vi "LabViewSLOTMACHINEFINAL.vi"() -> ()   [LabVIEW 2025]
panel:
  out "Bet info":string
  in  "stop":bool
  out "Minor Prize":bool
  out "Major Prize":bool
  out "Grand Prize":bool
  out "Array of Nums":dbl[](array[numeric])
  out "Balance Info":string
  out "Balance":i32
  in  "Bet Amount":i32
  in  "Spin":bool
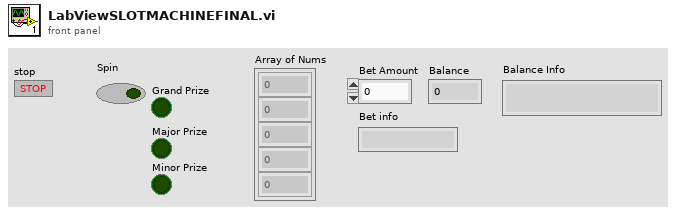
[diagram p1: front panel]
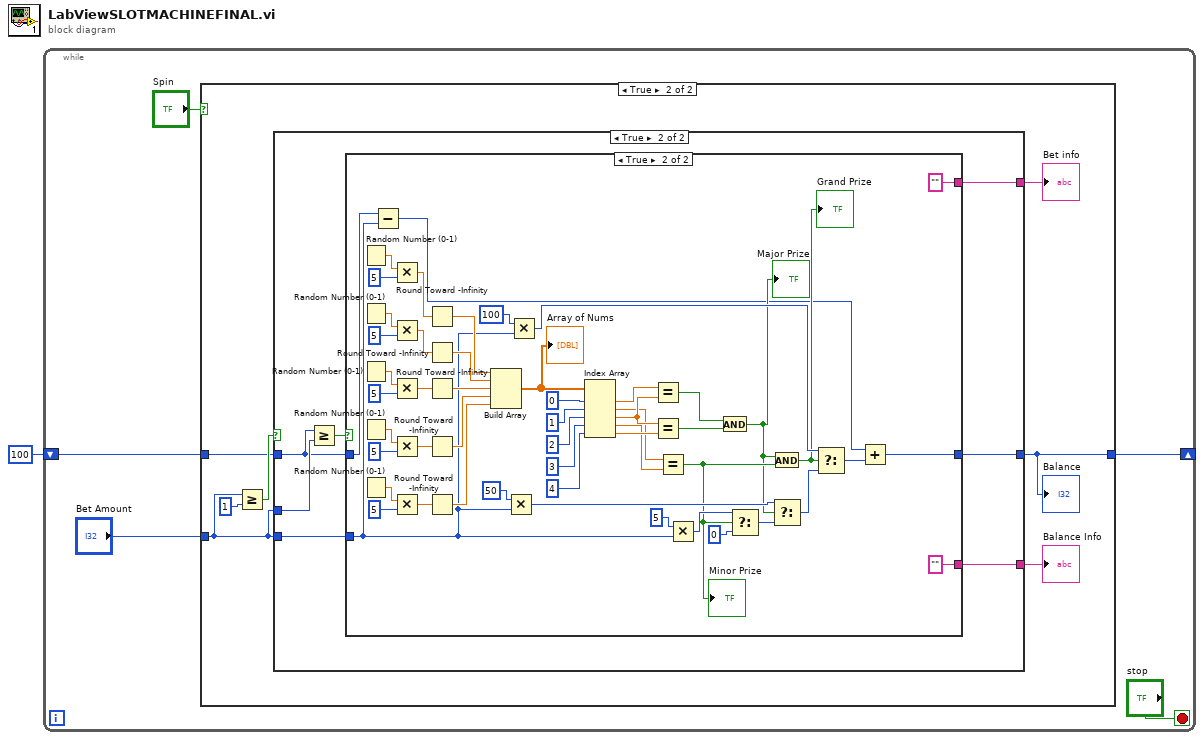
[diagram p0: block diagram]
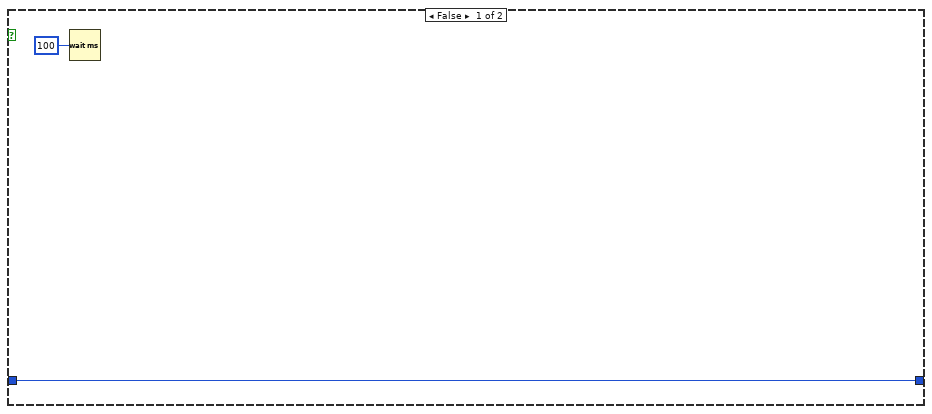
[diagram p2: hidden frame]
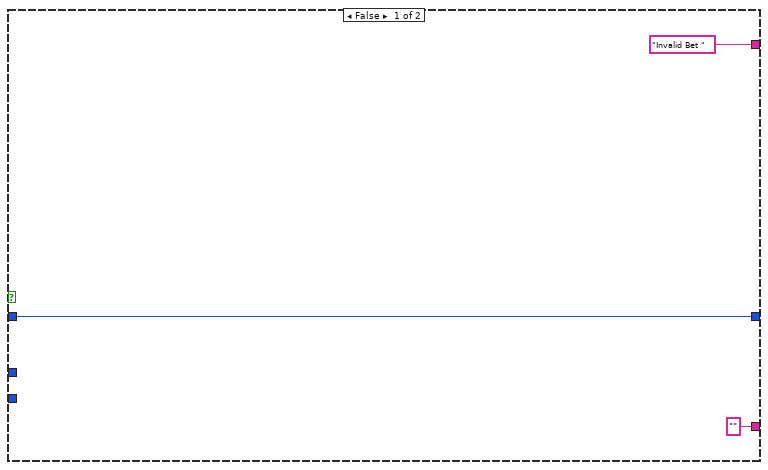
[diagram p3: hidden frame]
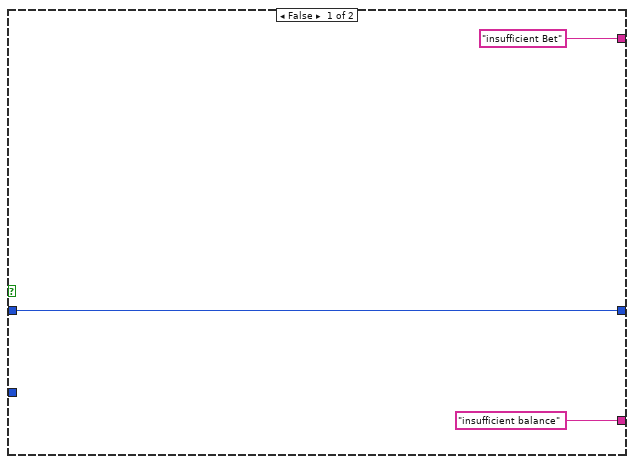
[diagram p4: hidden frame]
diagram:
  n1 = while {
    shift-right: [w6] -> _
    shift-left: 100 -> [w3]
    stop <- "stop" stop-if-true
    n2 = case shown="True" "Spin" {
      tunnel: w3 -> [w8 w13]
      tunnel: [w8 w12] -> w6
      tunnel: "Bet Amount" -> [_ w11]
      frame False {
        n3 = Wait (ms)(milliseconds to wait=100) -> ()  [unwired: 1 out]
      }
      frame True {
        n4 = Greater Or Equal?(x=w11, y=1) -> (x >= y?=w14:bool)
        n5 = case shown="True" w14 {
          tunnel: w11 -> [_ w25]
          tunnel: w13 -> [w18 w22]
          tunnel: [w18 w24] -> w12
          tunnel: w11 -> [_ w23]
          tunnel: ["" w20] -> w9
          tunnel: ["Invalid Bet " w19] -> w10
          frame False {
          }
          frame True {
            n6 = Greater Or Equal?(x=w22, y=w23) -> (x >= y?=w21:bool)
            n7 = case shown="True" w21 {
              tunnel: w25 -> [_ w43]
              tunnel: w22 -> [w28 w44]
              tunnel: [w28 w31] -> w24
              tunnel: ["insufficient balance" ""] -> w20
              tunnel: ["insufficient Bet" ""] -> w19
              frame False {
              }
              frame True {
                n8 = Random Number (0-1)() -> (number: 0 to 1=w75:dbl)
                n9 = Random Number (0-1)() -> (number: 0 to 1=w73:dbl)
                n10 = Random Number (0-1)() -> (number: 0 to 1=w71:dbl)
                n11 = Random Number (0-1)() -> (number: 0 to 1=w69:dbl)
                n12 = Random Number (0-1)() -> (number: 0 to 1=w67:dbl)
                n13 = Subtract(x=w44, y=w43) -> (x-y=w32:i32)
                n14 = Multiply(x=w75, y=5) -> (x*y=w74:dbl)
                n15 = Multiply(x=w73, y=5) -> (x*y=w72:dbl)
                n16 = Multiply(x=w71, y=5) -> (x*y=w70:dbl)
                n17 = Multiply(x=w69, y=5) -> (x*y=w68:dbl)
                n18 = Multiply(x=w67, y=5) -> (x*y=w66:dbl)
                n19 = Round Toward -Infinity(1:w74) -> (0:w80:dbl)
                n20 = Round Toward -Infinity(1:w72) -> (0:w79:dbl)
                n21 = Round Toward -Infinity(1:w70) -> (0:w78:dbl)
                n22 = Round Toward -Infinity(1:w68) -> (0:w77:dbl)
                n23 = Round Toward -Infinity(1:w66) -> (0:w76:dbl)
                n24 = Build Array(w80, w79, w78, w77, w76) -> (w62:dbl[])
                "Array of Nums" <- w62
                n25 = Multiply(x=50, y=w43) -> (x*y=w46:i32)
                n26 = Multiply(x=100, y=w43) -> (x*y=w45:i32)
                n27 = Index Array(array=w62, index #1=0, index #2=1, index #3=2, index #4=3, index #5=4) -> (element #1=w42:dbl, element #2=w37:dbl, element #3=w41:dbl, element #4=w36:dbl, element #5=w40:dbl)
                n28 = Equal?(x=w42, y=w41) -> (x = y?=w39:bool)
                n29 = Equal?(x=w41, y=w40) -> (x = y?=w38:bool)
                n30 = Equal?(x=w37, y=w36) -> (x = y?=w34:bool)
                "Minor Prize" <- w34
                n31 = Multiply(x=5, y=w43) -> (x*y=w47:i32)
                n32 = And(x=w39, y=w38) -> (x .and. y?=w33:bool)
                "Major Prize" <- w33
                n33 = Select(t=w47, s=w34, f=0) -> (s? t:f=w64:i32)
                n34 = And(x=w33, y=w34) -> (x .and. y?=w35:bool)
                "Grand Prize" <- w35
                n35 = Select(t=w46, s=w33, f=w64) -> (s? t:f=w63:i32)
                n36 = Select(t=w45, s=w35, f=w63) -> (s? t:f=w65:i32)
                n37 = Add(x=w32, y=w65) -> (x+y=w31:i32)
              }
            }
          }
        }
        "Balance" <- w12
        "Balance Info" <- w9
        "Bet info" <- w10
      }
    }
  }
